vi "Examples ZoomAndOffset.vi"() -> ()   [LabVIEW 2020, in "LcPictureBox.lvclass"]
uses:
  LcPictureBox.lvclass
  Pen.ctl
  Font.ctl
  <vilib>/picture/picture.llb/imagedata.ctl
  CallBackVIs/CallBAck_MouseDown.vi
  CallBackVIs/CallBack_MouseUp.vi
  CallBackVIs/CallBack_MouseMove.vi
  System.Windows.Forms
panel:
  in  "Origin":cluster{"x":sgl, "y":sgl}
  out "MouseUp":cluster{"X":i32, "Y":i32, "Button":i32}
  out "MouseDown":cluster{"X":i32, "Y":i32, "Button":i32}
  out "MouseMove":cluster{"X":i32, "Y":i32, "Button":i32}
  in  "Scale":sgl=0.1 min=0.1 max=10 step=0.5
  out "Error Out":errorcluster
  in  "PictureBox":refnum<k24>(container)
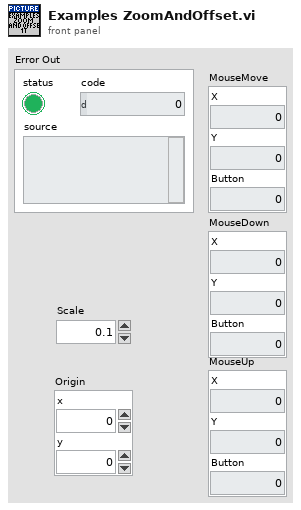
[diagram p1: front panel]
types:
  T1 = typedef "imagedata.ctl" = cluster{"image type":i32, "image depth":i32, "image":u8[], "mask":u8[], "colors":u32[], "Rectangle":cluster{"left":i16, "top":i16, "right":i16, "bottom":i16}}
  T2 = typedef "LcPictureBox.lvclass/Pen.ctl" = cluster{"Width":u16, "Style":enum32{"Solid", "Dash", "Dot", "DashDot", "DashDotDot"}}
  T3 = cluster{"horizontal":enum16{"Left", "Center", "Right"}, "vertical":enum16{"Top", "Center", "Bottom"}}
  T4 = typedef "LcPictureBox.lvclass/Font.ctl" = cluster{"FontName":string, "Size(Pts)":dbl, "Style":enum16{"Regular", "Bold", "Italic", "Underline", "Strikeout"}}
  T5 = cluster{"X":sgl, "Y":sgl, "Width":sgl, "Height":sgl}
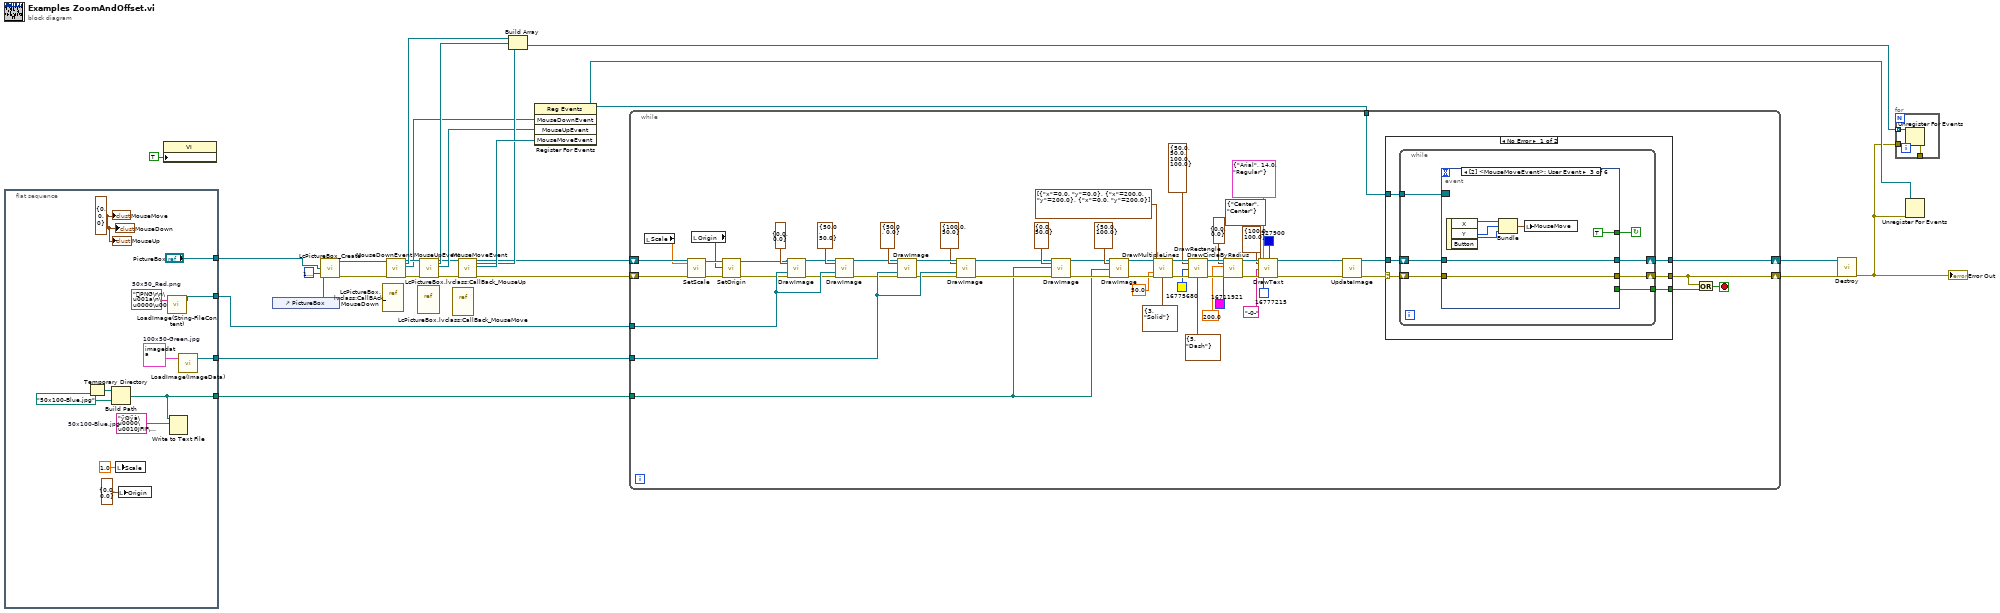
[diagram p0: block diagram]
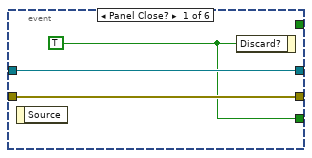
[diagram p2: hidden frame]
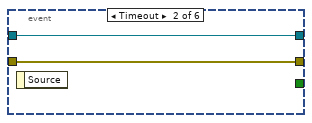
[diagram p3: hidden frame]
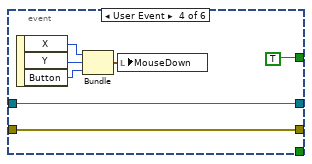
[diagram p4: hidden frame]
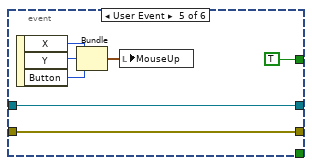
[diagram p5: hidden frame]
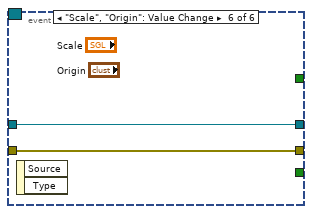
[diagram p6: hidden frame]
diagram:
  n1 = flat-sequence {
    tunnel: [w38] -> w26
    tunnel: [w37] -> w25
    tunnel: ["PictureBox"] -> w12
    tunnel: [w30] -> w4
    frame #0 {
      w29 = cluster{"X":i32, "Y":i32, "Button":i32} {"X"=0, "Y"=0, "Button"=0} ("MouseInfo")
      w31 = T1 {"image type"=0, "image depth"=24, "image"=array[15000 elements], "mask"=[], "colors"=[], "Rectangle"={"left"=0, "top"=0, "right"=100, "bottom"=50}}  # 100x50-Green.jpg
      w32 = "PNG\r\n\u001a\n\u0000\u0000\u0000\rIHDR\u0000\u0000\u00002\u0000\u0000\u00002\b\u0006\u0000\u0000\u0000\u001e?±\u0000\u0000\u0000\u0001sRGB\u0000®Î\u001cé\u0000\u0000\u0000\u0004gAMA\u0000\u0000±\u000büa\u0005\u0000\u0000\u0000\tpHYs\u0000\u0000\u000eÄ\u0000\u0000\u000eÄ\u0001+\u000e\u001b\u0000\u0000\u0002IDAThCí1kÛ@\u0018ß\u0016I\bä\u0018Å\u0016M\u0003b\u001a:tþA¡¦ £Wgèbºeö¥C¼zÌÖ©dÈ?ÈÞ¡¤ ­p\"ú°\u0005íw§S­Z\u0004Û­k¸\u0007ÌY§;½zï¾ï;\u001fÝ´ö~â\u0001ðX¶ÿ=Újh#ª¡¨6¢\u001aÚjh#ª¡¨6¢\u001aÚj³§1:_'¸9]o\u000fÇ¶¼ ÆIÃÉ\u001cg£ëîà¸f«µ¨Xçþ\u001d±êè:Ï\u000bCösèáûüá4fàyèZ\tFñ\u0015:Ó¹\u001c°\u0001\u0015éw&7iòòÊ,c\u0018^áhVÇië\t^>~p\u0011}+¨Xgó\u001cI\u0019>Ì¨uÂ\u001c¼qx;ÃeJá0\rÐ\f.Ñ¸ËÉûÖÞµ5tS>\u001b\u0018MèEøË\u0004\u0001úIAîóxõM+»<7ù²&øL\u0002íÚ\u000e\u0006ü60\u0014\fïãÂÈÃï*twÄ¨QBíâbràØðiÒh²iüè5<1÷è;Ãù4¢p°1h¸hË\u0011Õè,(\u0019iÛ.U\u0005ÚNj{Û-=å/\u0004\\ü`\u0018gCÖÃpqâÒê±k\u001cÐnøTmzD®LG²:G\f\u0013/åWaeó,4r¾Ì)thÕÿ¨:ð:«¤s|â­ifa\u000b2\n\u0019Þ\n\u0018>ò¼¶jx\u000bÐ9qÈóÂÙ¥Ð¡\u0017¿É|¹¿ÕG\u0001:QaB\u001f..."  # 50x50_Red.png
      w35 = "ÿØÿà\u0000\u0010JFIF\u0000\u0001\u0001\u0001\u0000`\u0000`\u0000\u0000ÿá\u0000fExif\u0000\u0000MM\u0000*\u0000\u0000\u0000\b\u0000\u0006\u0001\u0012\u0000\u0003\u0000\u0000\u0000\u0001\u0000\u0001\u0000\u0000\u0003\u0001\u0000\u0005\u0000\u0000\u0000\u0001\u0000\u0000\u0000V\u0003\u0003\u0000\u0001\u0000\u0000\u0000\u0001\u0000\u0000\u0000\u0000Q\u0010\u0000\u0001\u0000\u0000\u0000\u0001\u0001\u0000\u0000\u0000Q\u0011\u0000\u0004\u0000\u0000\u0000\u0001\u0000\u0000\u000eÃQ\u0012\u0000\u0004\u0000\u0000\u0000\u0001\u0000\u0000\u000eÃ\u0000\u0000\u0000\u0000\u0000\u0001 \u0000\u0000±ÿÛ\u0000C\u0000\u0002\u0001\u0001\u0002\u0001\u0001\u0002\u0002\u0002\u0002\u0002\u0002\u0002\u0002\u0003\u0005\u0003\u0003\u0003\u0003\u0003\u0006\u0004\u0004\u0003\u0005\u0007\u0006\u0007\u0007\u0007\u0006\u0007\u0007\b\t\u000b\t\b\b\n\b\u0007\u0007\n\r\n\n\u000b\f\f\f\f\u0007\t\u000e\u000f\r\f\u000e\u000b\f\f\fÿÛ\u0000C\u0001\u0002\u0002\u0002\u0003\u0003\u0003\u0006\u0003\u0003\u0006\f\b\u0007\b\f\f\f\f\f\f\f\f\f\f\f\f\f\f\f\f\f\f\f\f\f\f\f\f\f\f\f\f\f\f\f\f\f\f\f\f\f\f\f\f\f\f\f\f\f\f\f\f\f\fÿÀ\u0000\u0011\b\u0000d\u00002\u0003\u0001\"\u0000\u0002\u0011\u0001\u0003\u0011\u0001ÿÄ\u0000\u001f\u0000\u0000\u0001\u0005\u0001\u0001\u0001\u0001\u0001\u0001\u0000\u0000\u0000\u0000\u0000\u0000\u0000\u0000\u0001\u0002\u0003\u0004\u0005\u0006\u0007\b\t\n\u000bÿÄ\u0000µ\u0010\u0000\u0002\u0001\u0003\u0003\u0002\u0004\u0003\u0005\u0005\u0004\u0004\u0000\u0000\u0001}\u0001\u0002\u0003\u0000\u0004\u0011\u0005\u0012!1A\u0006\u0013Qa\u0007\"q\u00142¡\b#B±Á\u0015RÑð$3br\t\n\u0016\u0017\u0018\u0019\u001a%&'()*456789:CDEFGHIJSTUVWXYZcdefghijstuvwxyz¢£¤¥¦§¨©ª²³´µ¶·¸¹ºÂÃÄÅÆÇÈÉÊÒÓÔÕÖ×ØÙÚáâãäåæçèéêñòóôõö÷øùúÿÄ\u0000\u001f\u0001\u0000\u0003\u0001\u0001\u0001\u0001\u0001\u0001\u0001\u0001\u0001\u0000\u0000\u0000\u0000\u0000\u0000\u0001\u0002\u0003\u0004\u0005\u0006\u0007\b\t\n\u000bÿÄ\u0000µ\u0011\u0000\u0002\u0001\u0002\u0004\u0004\u0003\u0004\u0007\u0005\u0004\u0004\u0000\u0001\u0002w\u0000\u0001\u0002\u0003\u0011\u0004\u0005!1\u0006\u0012AQ\u0007aq\u0013\"2\b\u0014B¡±Á\t#3Rð\u0015brÑ\n\u0016$4á%ñ\u0017\u0018\u0019\u001a&'..."  # 50x100-Blue.jpg
      n2 = Temporary Directory() -> (w34:path)
      n3 = Build Path(base path=w34, name or relative path=path "50x100-Blue.jpg" ("Filename")) -> (appended path=w30:path)
      n4 = local write "Scale"(sgl 1.0 ("Scale")) -> ()
      n5 = local write "Origin"(cluster{"x":sgl, "y":sgl} {"x"=0.0, "y"=0.0} ("Origin")) -> ()
      n6 = call "LoadImage(String-FileContent).vi"("ImageFileContent"=w32) -> ("ImageOut"=w38:refnum<k24>)  [unwired: 16 in, 2 out]
      n7 = Write to Text File(file (use dialog)=w30, text=w35) -> ()  [unwired: 2 in, 3 out]
      n8 = call "LoadImage(ImageData).vi"("image data"=w31) -> ("ImageOut"=w37:refnum<k24>)  [unwired: 16 in, 2 out]
      "MouseMove" <- w29
      "MouseDown" <- w29
      "MouseUp" <- w29
    }
  }
  n9 = property class="VI"("Front Panel.IsFrontmost"=TRUE ("Front Panel Window:Is Frontmost")) -> ()  [unwired: 2 in, 2 out]
  n10 = control-ref of="PictureBox"() -> (w11:refnum<vi>)
  n11 = call "LcPictureBox_Create.vi"("PictureBox"=w12, "PictureBoxActiveXReference"=w11, "BgColor(None)"=u32 16777216) -> ("reference out"=w23:refnum<class "LcPictureBox.lvclass">, "Error Out"=w24:errorcluster)  [unwired: 14 in, 1 out]
  n12 = vi-ref "LcPictureBox.lvclass:CallBAck_MouseDown.vi"() -> ()  [unwired: 1 out]
  n13 = call-dynamic "MouseDownEvent.vi"("reference in"=w23, "error in (no error)"=w24) -> ("reference out"=w14:refnum<class "LcPictureBox.lvclass">, "Event Callback Refnum"=w19:refnum<k27>, "MouseDownEvent"=w13:refnum<user-event>, "error out"=w16:errorcluster)  [unwired: 14 in]
  n14 = vi-ref "LcPictureBox.lvclass:CallBack_MouseUp.vi"() -> ()  [unwired: 1 out]
  n15 = call-dynamic "MouseUpEvent.vi"("reference in"=w14, "error in (no error)"=w16) -> ("reference out"=w15:refnum<class "LcPictureBox.lvclass">, "Event Callback Refnum"=w20:refnum<k27>, "MouseUpEvent"=w17:refnum<user-event>, "error out"=w18:errorcluster)  [unwired: 14 in]
  n16 = vi-ref "LcPictureBox.lvclass:CallBack_MouseMove.vi"() -> ()  [unwired: 1 out]
  n17 = call-dynamic "MouseMoveEvent.vi"("reference in"=w15, "error in (no error)"=w18) -> ("reference out"=w9:refnum<class "LcPictureBox.lvclass">, "Event Callback Refnum"=w21:refnum<k27>, "MouseMoveEvent"=w22:refnum<user-event>, "error out"=w3:errorcluster)  [unwired: 14 in]
  n18 = Build Array(w19, w20, w21) -> (w7:refnum<k27>[])
  n19 = register-events(w13, w17, w22) -> (reference out=w8:refnum<event-registration>)  [unwired: 2 in, 1 out]
  n20 = while {
    tunnel: w26 -> [w97]
    tunnel: w25 -> [w96]
    tunnel: w8 -> [w94]
    tunnel: w4 -> [w75]
    shift-right: [w93] -> w6
    shift-left: w9 -> [w95]
    shift-right: [w72] -> w2
    shift-left: w3 -> [w73]
    stop <- w70 stop-if-true
    n21 = local read "Scale"() -> (w42:sgl)
    n22 = call-dynamic "SetScale.vi"("reference in"=w95, "ScaleFactor"=w42, "Error In"=w73) -> ("reference out"=w46:refnum<class "LcPictureBox.lvclass">, "Error Out"=w45:errorcluster)  [unwired: 15 in]
    n23 = local read "Origin"() -> (w41:cluster{"x":sgl, "y":sgl})
    n24 = call-dynamic "SetOrigin.vi"("reference in"=w46, "Origin"=w41, "Error In"=w45) -> ("reference out"=w43:refnum<class "LcPictureBox.lvclass">, "Error Out"=w44:errorcluster)  [unwired: 15 in]
    n25 = call-dynamic "DrawImage.vi"("reference in"=w43, "UpperLeftCorner(0,0)"=cluster{"x":sgl, "y":sgl} {"x"=0.0, "y"=0.0} ("UpperLeftCorner"), "Image"=w97, "Error In"=w44) -> ("reference out"=w83:refnum<class "LcPictureBox.lvclass">, "Error Out"=w82:errorcluster)  [unwired: 14 in]
    n26 = call-dynamic "DrawImage.vi"("reference in"=w83, "UpperLeftCorner(0,0)"=cluster{"x":sgl, "y":sgl} {"x"=50.0, "y"=50.0} ("UpperLeftCorner"), "Image"=w97, "Error In"=w82) -> ("reference out"=w87:refnum<class "LcPictureBox.lvclass">, "Error Out"=w88:errorcluster)  [unwired: 14 in]
    n27 = call-dynamic "DrawImage.vi"("reference in"=w87, "UpperLeftCorner(0,0)"=cluster{"x":sgl, "y":sgl} {"x"=50.0, "y"=0.0} ("UpperLeftCorner"), "Image"=w96, "Error In"=w88) -> ("reference out"=w86:refnum<class "LcPictureBox.lvclass">, "Error Out"=w85:errorcluster)  [unwired: 14 in]
    n28 = call-dynamic "DrawImage.vi"("reference in"=w86, "UpperLeftCorner(0,0)"=cluster{"x":sgl, "y":sgl} {"x"=100.0, "y"=50.0} ("UpperLeftCorner"), "Image"=w96, "Error In"=w85) -> ("reference out"=w77:refnum<class "LcPictureBox.lvclass">, "Error Out"=w76:errorcluster)  [unwired: 14 in]
    n29 = call-dynamic "DrawImage.vi"("reference in"=w77, "UpperLeftCorner(0,0)"=cluster{"x":sgl, "y":sgl} {"x"=0.0, "y"=50.0} ("UpperLeftCorner"), "Filename"=w75, "Error In"=w76) -> ("reference out"=w79:refnum<class "LcPictureBox.lvclass">, "Error Out"=w80:errorcluster)  [unwired: 14 in]
    n30 = call-dynamic "DrawImage.vi"("reference in"=w79, "UpperLeftCorner(0,0)"=cluster{"x":sgl, "y":sgl} {"x"=50.0, "y"=100.0} ("UpperLeftCorner"), "Filename"=w75, "Error In"=w80) -> ("reference out"=w63:refnum<class "LcPictureBox.lvclass">, "Error Out"=w62:errorcluster)  [unwired: 14 in]
    n31 = call-dynamic "DrawMultipleLines.vi"("reference in"=w63, "LineEndPoints"=cluster{"x":dbl, "y":dbl}[] [{"x"=0.0, "y"=0.0}, {"x"=200.0, "y"=200.0}, {"x"=0.0, "y"=200.0}], "Alpha(100%)"=50.0, "Error In"=w62, "Pen(Width=1, Solid)"=T2 {"Width"=3, "Style"=enum."Solid"}) -> ("reference out"=w69:refnum<class "LcPictureBox.lvclass">, "Error Out"=w68:errorcluster)  [unwired: 13 in]
    n32 = call-dynamic "DrawRectangle.vi"("reference in"=w69, "Rectangle"=T5 {"X"=50.0, "Y"=50.0, "Width"=100.0, "Height"=100.0}, "Color(Black)"=u32 16775680, "Error In"=w68, "Pen(Width=1, Solid)"=T2 {"Width"=5, "Style"=enum."Dash"}) -> ("reference out"=w67:refnum<class "LcPictureBox.lvclass">, "Error Out"=w66:errorcluster)  [unwired: 13 in]
    n33 = call-dynamic "DrawCircleByRadius.vi"("reference in"=w67, "Center"=cluster{"x":sgl, "y":sgl} {"x"=0.0, "y"=0.0}, "Radius"=sgl 200.0, "Color(Black)"=u32 16711921, "Error In"=w66) -> ("reference out"=w65:refnum<class "LcPictureBox.lvclass">, "Error Out"=w64:errorcluster)  [unwired: 13 in]
    n34 = call-dynamic "DrawText.vi"("reference in"=w65, "Origin"=cluster{"X":sgl, "Y":sgl} {"X"=100.0, "Y"=100.0}, "Alignment(Left,Top)"=T3 {"horizontal"=enum."Center", "vertical"=enum."Center"}, "Text"="-0-", "Error In"=w64, "Font(Arial,14pts,Regular)"=T4 {"FontName"="Arial", "Size(Pts)"=14.0, "Style"=enum."Regular"}, "Color(Black)"=u32 16777215 ("BgColor(Transparent)"), "BgColor(Transparent)"=u32 327900) -> ("reference out"=w61:refnum<class "LcPictureBox.lvclass">, "Error Out"=w60:errorcluster)  [unwired: 10 in]
    n35 = call-dynamic "UpdateImage.vi"("reference in"=w61, "Error In"=w60) -> ("reference out"=w91:refnum<class "LcPictureBox.lvclass">, "Error Out"=w92:errorcluster)  [unwired: 14 in, 2 out]
    n36 = case shown="No Error" w92 {
      selector: w92 -> [w103 w140]
      tunnel: w91 -> [w102 w139]
      tunnel: w94 -> [w101 _]
      tunnel: [w100 w140] -> w72
      tunnel: [w99 w139] -> w93
      tunnel: [w98 _] -> w71
      frame No Error {
        n37 = while {
          tunnel: w101 -> [w108]
          shift-right: [w107] -> w100
          shift-left: w103 -> [w110]
          shift-right: [w106] -> w99
          shift-left: w102 -> [w109]
          tunnel: [w104] -> w98
          stop <- w105 continue-if-true
          n38 = event shown="[2] <MouseMoveEvent>: User Event" {
            selector: w108 -> [_ _ _ _ _ _]
            dyn-events: _ -> [_ _ _ _ _ _]
            timeout: _ -> [_ _ _ _ _ _]
            tunnel: w110 -> [w113 w114 w121 w128 w135 w137]
            tunnel: [w113 w114 w121 w128 w135 w137] -> w107
            tunnel: w109 -> [w112 w115 w122 w129 w136 w138]
            tunnel: [w112 w115 w122 w129 w136 w138] -> w106
            tunnel: [_ _ TRUE TRUE TRUE _] -> w105
            tunnel: [w111 _ _ _ _ _] -> w104
            event Panel Close? {
              w111 = TRUE ("Discard?")
              n39 = event-data() -> ()  [unwired: 1 in, 1 out]
              n40 = event-data("Discard?"=w111) -> ()  [unwired: 1 in, 1 out]
            }
            event Timeout {
              n41 = event-data() -> ()  [unwired: 1 in, 1 out]
            }
            event User Event {
              n42 = event-data() -> ("X"=w119:i32, "Y"=w118:i32, "Button"=w117:i32)  [unwired: 1 in]
              n43 = Bundle("X"=w119, "Y"=w118, "Button"=w117) -> (w116:cluster{"X":i32, "Y":i32, "Button":i32})  [unwired: 1 in]
              n44 = local write "MouseMove"(w116) -> ()
            }
            event User Event {
              n45 = event-data() -> ("X"=w125:i32, "Y"=w126:i32, "Button"=w124:i32)  [unwired: 1 in]
              n46 = Bundle("X"=w125, "Y"=w126, "Button"=w124) -> (w127:cluster{"X":i32, "Y":i32, "Button":i32})  [unwired: 1 in]
              n47 = local write "MouseDown"(w127) -> ()
            }
            event User Event {
              n48 = event-data() -> ("X"=w133:i32, "Y"=w132:i32, "Button"=w131:i32)  [unwired: 1 in]
              n49 = Bundle("X"=w133, "Y"=w132, "Button"=w131) -> (w134:cluster{"X":i32, "Y":i32, "Button":i32})  [unwired: 1 in]
              n50 = local write "MouseUp"(w134) -> ()
            }
            event "Scale", "Origin": Value Change {
              n51 = event-data() -> ()  [unwired: 1 in, 2 out]
            }
          }
        }
      }
      frame Error {
      }
    }
    n52 = Or(x=w72, y=w71) -> (x .or. y?=w70:bool)
  }
  n53 = call-dynamic "Destroy.vi"("reference in"=w6, "Error In"=w2) -> ("Error Out"=w1:errorcluster)  [unwired: 16 in, 1 out]
  "Error Out" <- w1
  n54 = for {
    tunnel: w7 -> [w143] mode=indexing
    tunnel: [w142] -> _
    tunnel: w1 -> [w141]
    n55 = Unregister For Events(event registration refnum=w143, error in=w141) -> (error out=w142:errorcluster)
  }
  n56 = Unregister For Events(event registration refnum=w8, error in=w1) -> ()  [unwired: 1 out]
